vi "Down Heap.vi"(8 "error in (no error)":errorcluster, 10 "index":i32, 11 "Astar Open List in":refnum<class "NI_Robotics_Priority Queue.lvclass">) -> (0 "error out":errorcluster, 3 "Astar Open List out":refnum<class "NI_Robotics_Priority Queue.lvclass">)   [LabVIEW 2017, in "NI_Robotics_Priority Queue.lvclass"]
uses:
  <vilib>/robotics/Navigation/shared/Priority Queue/NI_Robotics_Priority Queue.lvclass
  <vilib>/robotics/Navigation/shared/Priority Queue/NI_Robotics_Priority Queue.lvclass/NI_Robotics_Priority Queue.ctl
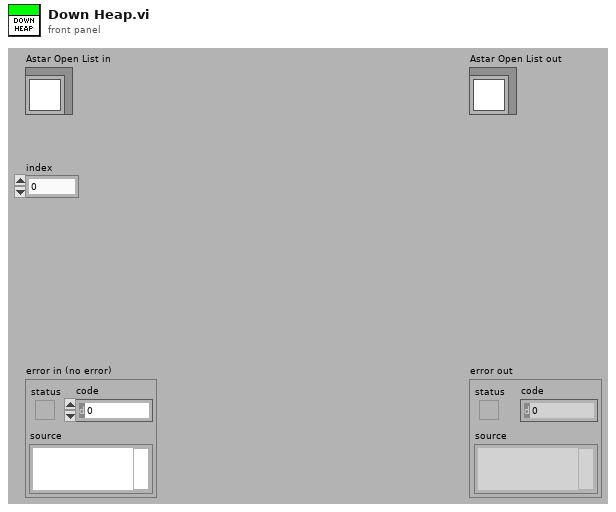
[diagram p1: front panel]
types:
  T1 = typedef "NI_Robotics_Priority Queue.lvclass/Open List Element.ctl" = cluster{"f":dbl, "g":dbl, "node Ref":refnum<data-value>}
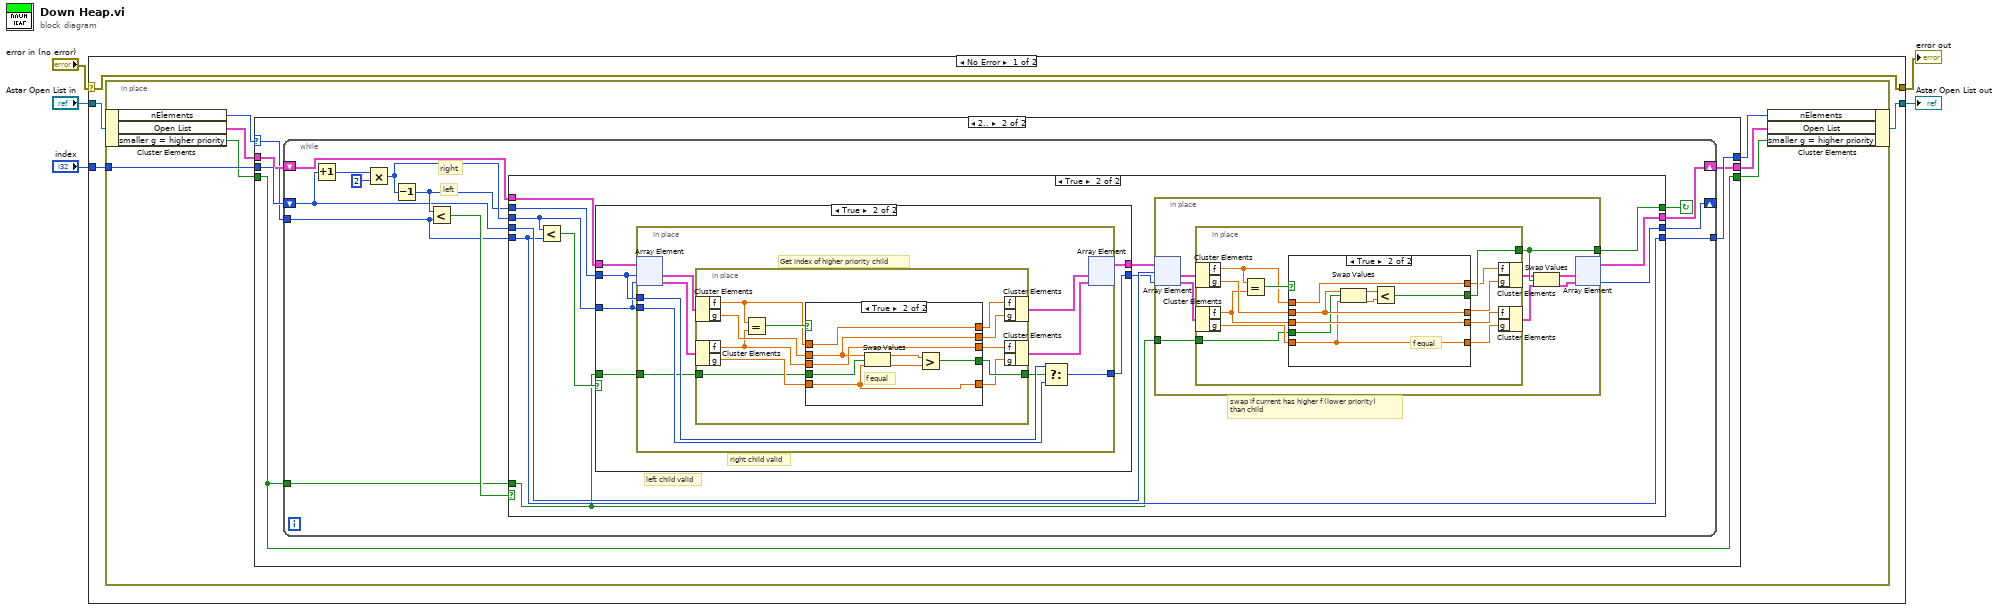
[diagram p0: block diagram]
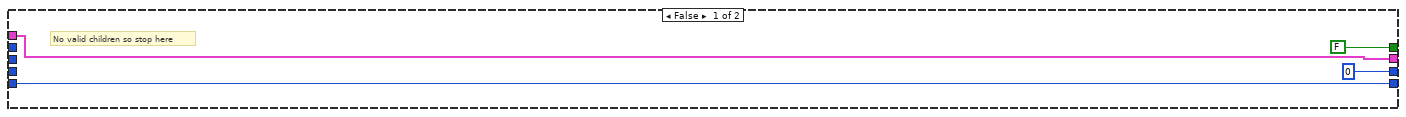
[diagram p3: hidden frame]
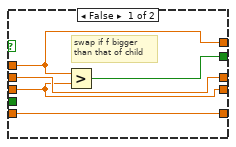
[diagram p4: hidden frame]
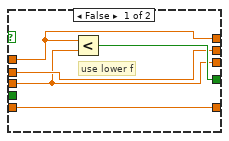
[diagram p6: hidden frame]
diagram:
  n1 = case shown="No Error" "error in (no error)" {
    selector: "error in (no error)" -> [w6 w129]
    tunnel: [w6 w129] -> w4
    tunnel: [w8 w128] -> w2
    tunnel: "Astar Open List in" -> [w9 w128]
    tunnel: "index" -> [w7 _]
    frame No Error {
      n2 = in-place {
        in-place-border: w7 -> [w16]
        n3 = in-place-cluster #1(w9) -> ("nElements"=w12:i32, "Open List"=w15:T1[], "smaller g = higher priority"=w11:bool)
        n4 = case shown="2.." w12 {
          selector: w12 -> [w18 w21]
          tunnel: w16 -> [_ w25]
          tunnel: w15 -> [w19 w24]
          tunnel: [w18 w23] -> w14
          tunnel: [w19 w22] -> w13
          tunnel: w11 -> [w17 w20]
          tunnel: [w17 w20] -> w10
          frame ..1 {
            # "One or less elements in the list. Do nothing"
          }
          frame 2.. {
            n5 = while {
              shift-right: [w28] -> _
              shift-left: w25 -> [w31]
              shift-right: [w30] -> w22
              shift-left: w24 -> [w33]
              tunnel: w21 -> [w32]
              tunnel: [w29] -> w23
              tunnel: w20 -> [w26]
              stop <- w27 continue-if-true
              # "right"
              # "left"
              n6 = Increment(x=w31) -> (x+1=w38:i32)
              n7 = Multiply(x=w38, y=2) -> (x*y=w36:i32)
              n8 = Decrement(x=w36) -> (x-1=w34:i32)
              n9 = Less?(x=w34, y=w32) -> (x < y?=w35:bool)
              n10 = case shown="True" w35 {
                tunnel: w34 -> [_ w52]
                tunnel: w36 -> [_ w51]
                tunnel: w33 -> [w41 w53]
                tunnel: w32 -> [w42 w46]
                tunnel: w31 -> [_ w49]
                tunnel: [w41 w47] -> w30
                tunnel: [w42 w46] -> w29
                tunnel: [FALSE w45] -> w27
                tunnel: [0 w44] -> w28
                tunnel: w26 -> [_ w43]
                frame False {
                  # "No valid children so stop here"
                }
                frame True {
                  # "swap if current has higher f (lower priority)\nthan child"
                  # "left child valid"
                  n11 = Less?(x=w51, y=w46) -> (x < y?=w54:bool)
                  n12 = case shown="True" w54 {
                    tunnel: w53 -> [w87 w94]
                    tunnel: w52 -> [w88 w93]
                    tunnel: w51 -> [_ w92]
                    tunnel: [w88 w91] -> w48
                    tunnel: [w87 w90] -> w50
                    tunnel: w43 -> [_ w89]
                    frame False {
                      # "use left child"
                      # "right child invalid"
                    }
                    frame True {
                      # "right child valid"
                      n13 = in-place {
                        in-place-border: w93 -> [w103]
                        in-place-border: w92 -> [w102]
                        in-place-border: [w101] -> w91
                        in-place-border: w89 -> [w95]
                        # "Get index of higher priority child"
                        n14 = in-place-array #2(w94, w93, w92) -> (w99:T1, w98:T1)
                        n15 = in-place {
                          in-place-border: [w113] -> w100
                          in-place-border: w95 -> [w104]
                          n16 = in-place-cluster #3(w99) -> ("f"=w112:dbl, "g"=w111:dbl)
                          n17 = in-place-cluster #4(w98) -> ("f"=w110:dbl, "g"=w109:dbl)
                          n18 = Equal?(x=w112, y=w110) -> (x = y?=w114:bool)
                          n19 = case shown="True" w114 {
                            tunnel: w109 -> [w115 w124]
                            tunnel: w111 -> [w117 w123]
                            tunnel: w112 -> [w118 w126]
                            tunnel: w110 -> [w116 w125]
                            tunnel: [w119 w127] -> w113
                            tunnel: [w118 w126] -> w107
                            tunnel: [w117 w123] -> w108
                            tunnel: [w116 w125] -> w105
                            tunnel: [w115 w124] -> w106
                            tunnel: w104 -> [_ w122]
                            frame False {
                              # "use lower f"
                              n20 = Less?(x=w118, y=w116) -> (x < y?=w119:bool)
                            }
                            frame True {
                              # "f equal"
                              n21 = Swap Values(12:w123, 13:w122, 14:w124) -> (1:w121:dbl, 3:w120:dbl)
                              n22 = Greater?(x=w121, y=w120) -> (0:w127:bool)
                            }
                          }
                          n23 = in-place-cluster #3("f"=w107, "g"=w108) -> (w97:T1)
                          n24 = in-place-cluster #4("f"=w105, "g"=w106) -> (w96:T1)
                        }
                        n25 = Select(t=w103, s=w100, f=w102) -> (s? t:f=w101:i32)
                        n26 = in-place-array #2(w97, w96) -> (w90:T1[])  [unwired: 2 out]
                      }
                    }
                  }
                  n27 = in-place {
                    in-place-border: [w58] -> w45
                    in-place-border: w43 -> [w55]
                    n28 = in-place-array #5(w50, w49, w48) -> (w60:T1, w59:T1)
                    n29 = in-place {
                      in-place-border: [w72] -> w58
                      in-place-border: w55 -> [w63]
                      n30 = in-place-cluster #6(w60) -> ("f"=w71:dbl, "g"=w70:dbl)
                      n31 = in-place-cluster #7(w59) -> ("f"=w69:dbl, "g"=w68:dbl)
                      n32 = Equal?(x=w71, y=w69) -> (x = y?=w73:bool)
                      n33 = case shown="True" w73 {
                        tunnel: w68 -> [w74 w82]
                        tunnel: w70 -> [w76 w83]
                        tunnel: w71 -> [w77 w84]
                        tunnel: w69 -> [w75 w85]
                        tunnel: [w78 w86] -> w72
                        tunnel: [w74 w82] -> w67
                        tunnel: [w75 w85] -> w66
                        tunnel: [w76 w83] -> w65
                        tunnel: [w77 w84] -> w64
                        tunnel: w63 -> [_ w81]
                        frame False {
                          # "swap if f bigger\nthan that of child"
                          n34 = Greater?(x=w77, y=w75) -> (0:w78:bool)
                        }
                        frame True {
                          # "f equal"
                          n35 = Swap Values(12:w83, 13:w81, 14:w82) -> (1:w80:dbl, 3:w79:dbl)
                          n36 = Less?(x=w80, y=w79) -> (x < y?=w86:bool)
                        }
                      }
                      n37 = in-place-cluster #6("f"=w64, "g"=w65) -> (w56:T1)
                      n38 = in-place-cluster #7("f"=w66, "g"=w67) -> (w57:T1)
                    }
                    n39 = Swap Values(12:w56, 13:w58, 14:w57) -> (1:w61:T1, 3:w62:T1)
                    n40 = in-place-array #5(w61, w62) -> (w47:T1[], w44:i32)  [unwired: 1 out]
                  }
                }
              }
            }
          }
        }
        n41 = in-place-cluster #1("nElements"=w14, "Open List"=w13, "smaller g = higher priority"=w10) -> (w8:refnum<class "NI_Robotics_Priority Queue.lvclass">)
      }
    }
    frame Error {
    }
  }
  "error out" <- w4
  "Astar Open List out" <- w2
